vi "DriveBase.vi"(9 "Elevator State":string="Hatch_Rocket_1") -> ()   [LabVIEW 2018]
uses:
  RobotStates.vi
  Inputs_DriverStation.vi
  SensorReadings.vi
panel:
  in  "Forward Acceleration (p/s)":dbl=10.0
  in  "Time Above Speed (ms)":u32=100
  in  "Stabilization Height (in)":dbl=36.0
  in  "Switch to Low Gear (ft/s)":dbl=0.5
  in  "Switch to High Gear (ft/s)":dbl=5.0
  in  "Elevator Danger Height (in)":dbl=52.0
  in  "Backward Acceleration (p/s)":dbl=1.0
  in  "Climb-Drive Bias":dbl=-0.4
  in  "Turning Deadband":dbl=0.1
  in  "Throttle Deadband":dbl=0.2
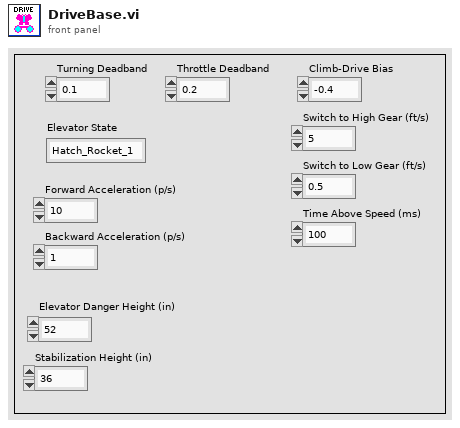
[diagram p1: front panel]
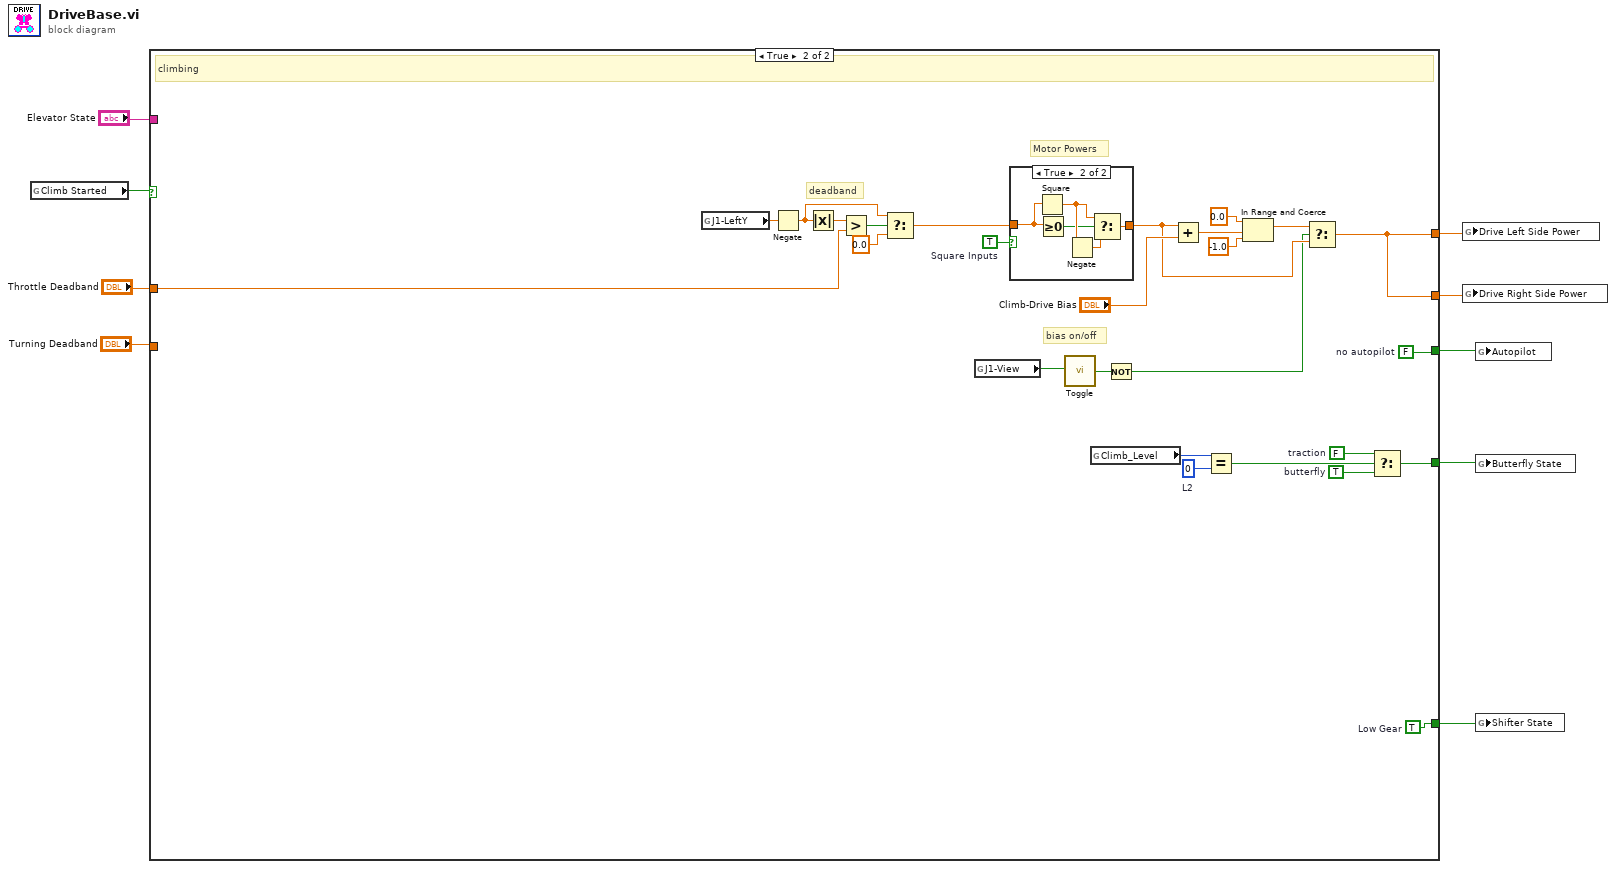
[diagram p0: block diagram]
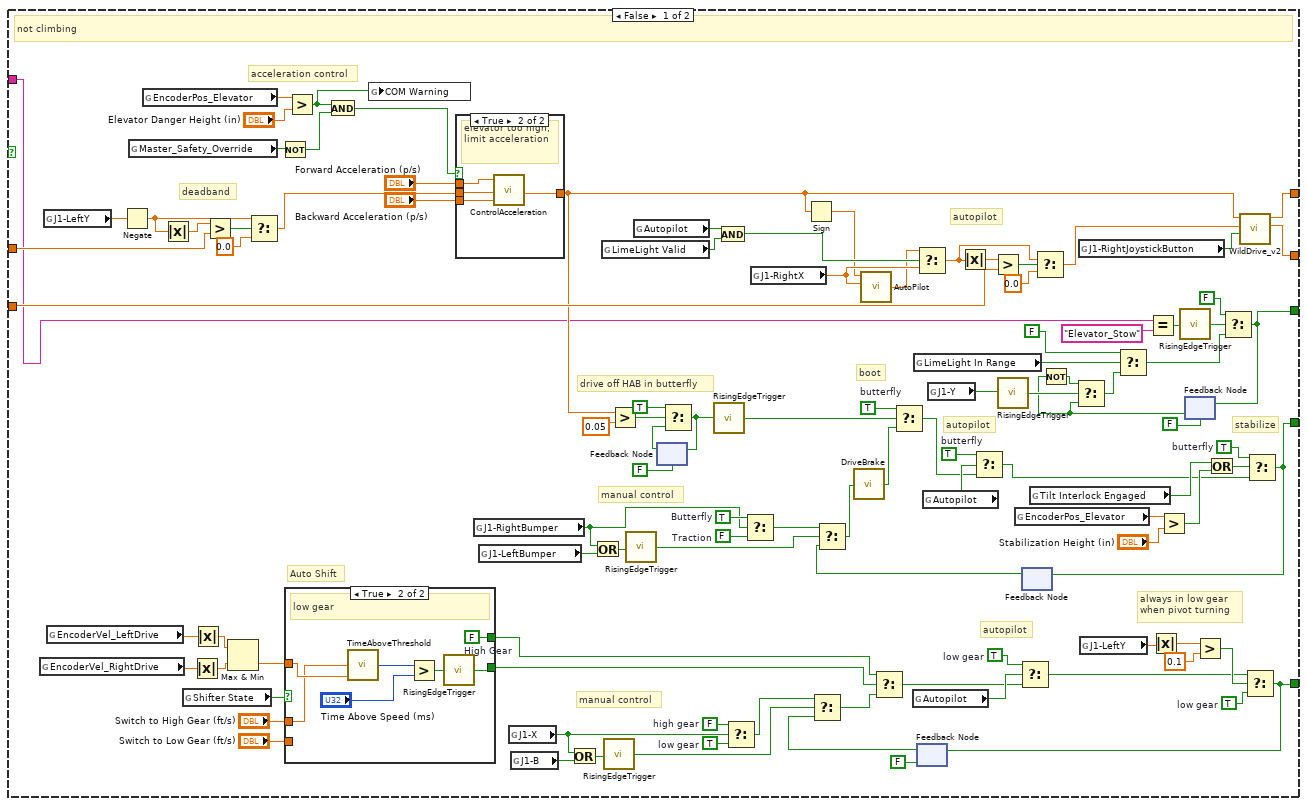
[diagram p2: hidden frame]
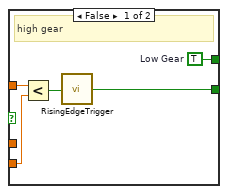
[diagram p3: hidden frame]
diagram:
  n1 = global read "RobotStates.vi" "Climb Started"() -> (w5:bool)
  n2 = case shown="True" w5 {
    tunnel: [w53 w137] -> w9
    tunnel: [w43 w157] -> w8
    tunnel: "Throttle Deadband" -> [w105 w149]
    tunnel: "Turning Deadband" -> [w104 _]
    tunnel: [w95 w139] -> w1
    tunnel: [w94 w139] -> w2
    tunnel: [w20 w138] -> w4
    tunnel: "Elevator State" -> [w19 _]
    frame False {
      w32 = TRUE  # butterfly
      w35 = TRUE  # low gear
      w42 = TRUE  # low gear
      w54 = FALSE  # Traction
      w55 = TRUE  # Butterfly
      w61 = TRUE  # butterfly
      w68 = TRUE  # butterfly
      w97 = TRUE  # low gear
      w98 = FALSE  # high gear
      # "deadband"
      # "acceleration control"
      # "always in low gear\nwhen pivot turning"
      # "autopilot"
      # "manual control"
      # "stabilize"
      # "autopilot"
      # "boot"
      # "manual control"
      # "autopilot"
      # "drive off HAB in butterfly"
      # "Auto Shift"
      # "not climbing"
      n3 = global read "SensorReadings.vi" "EncoderVel_RightDrive"() -> (w77:dbl)
      n4 = global read "Inputs_DriverStation.vi" "J1-LeftY"() -> (w110:dbl)
      n5 = global read "SensorReadings.vi" "EncoderVel_LeftDrive"() -> (w78:dbl)
      n6 = Negate(x=w110) -> (-x=w113:dbl)
      n7 = global read "Inputs_DriverStation.vi" "Master_Safety_Override"() -> (w83:bool)
      n8 = global read "SensorReadings.vi" "EncoderPos_Elevator"() -> (w86:dbl)
      n9 = Absolute Value(x=w113) -> (abs(x)=w108:dbl)
      n10 = global read "RobotStates.vi" "Shifter State"() -> (w76:bool)
      n11 = Absolute Value(x=w77) -> (abs(x)=w70:dbl)
      n12 = Absolute Value(x=w78) -> (abs(x)=w71:dbl)
      n13 = Greater?(x=w108, y=w105) -> (0:w109:bool)
      n14 = Max & Min(x=w71, y=w70) -> (min(x,y)=w49:dbl)  [unwired: 1 out]
      n15 = Select(t=w113, s=w109, f=0.0) -> (s? t:f=w88:dbl)
      n16 = Not(x=w83) -> (.not. x?=w82:bool)
      n17 = case shown="True" w76 {
        tunnel: w49 -> [w119 w121]
        tunnel: "Switch to High Gear (ft/s)" -> [_ w120]
        tunnel: "Switch to Low Gear (ft/s)" -> [w118 _]
        tunnel: [w115 w125] -> w69
        tunnel: [w117 w126] -> w72
        frame False {
          w117 = TRUE  # Low Gear
          # "high gear"
          n18 = Less?(x=w119, y=w118) -> (x < y?=w116:bool)
          n19 = call "RisingEdgeTrigger.vi"("Raw Signal"=w116) -> ("Trigger"=w115:bool)
        }
        frame True {
          w126 = FALSE  # High Gear
          # "low gear"
          n20 = call "TimeAboveThreshold.vi"("Current Value"=w121, "Threshold"=w120) -> ("Time Above"=w124:u32)  [unwired: 3 in]
          n21 = Greater?(x=w124, y="Time Above Speed (ms)") -> (0:w122:bool)
          n22 = call "RisingEdgeTrigger.vi"("Raw Signal"=w122) -> ("Trigger"=w125:bool)
        }
      }
      n23 = Greater?(x=w86, y="Elevator Danger Height (in)") -> (0:w79:bool)
      n24 = And(x=w79, y=w82) -> (x .and. y?=w84:bool)
      n25 = global write "RobotStates.vi" "COM Warning"(w79) -> ()
      n26 = case shown="True" w84 {
        tunnel: w88 -> [w127 w131]
        tunnel: [w127 w130] -> w29
        tunnel: "Backward Acceleration (p/s)" -> [_ w129]
        tunnel: "Forward Acceleration (p/s)" -> [_ w128]
        frame False {
          # "elevator down"
        }
        frame True {
          # "elevator too high, limit acceleration"
          n27 = call "ControlAcceleration.vi"("Backward Acceleration (p/s)"=w129, "Raw"=w131, "Forward Acceleration (p/s)"=w128) -> ("Controlled"=w130:dbl)
        }
      }
      n28 = global read "Inputs_DriverStation.vi" "J1-RightBumper"() -> (w51:bool)
      n29 = global read "Inputs_DriverStation.vi" "J1-LeftBumper"() -> (w52:bool)
      n30 = global read "Inputs_DriverStation.vi" "J1-X"() -> (w44:bool)
      n31 = global read "Inputs_DriverStation.vi" "J1-B"() -> (w102:bool)
      n32 = Or(x=w44, y=w102) -> (x .or. y?=w103:bool)
      n33 = Or(x=w51, y=w52) -> (x .or. y?=w59:bool)
      n34 = global read "SensorReadings.vi" "LimeLight Valid"() -> (w89:bool)
      n35 = call "RisingEdgeTrigger.vi"("Raw Signal"=w103) -> ("Trigger"=w99:bool)
      n36 = Greater?(x=w29, y=0.05) -> (0:w63:bool)
      n37 = call "RisingEdgeTrigger.vi"("Raw Signal"=w59) -> ("Trigger"=w56:bool)
      n38 = global read "RobotStates.vi" "Autopilot"() -> (w91:bool)
      n39 = feedback #1(FALSE) -> (w66:bool)
      n40 = Select(t=TRUE, s=w63, f=w66) -> (s? t:f=w65:bool)
      n41 = feedback-in #1(w65) -> ()
      n42 = call "RisingEdgeTrigger.vi"("Raw Signal"=w65) -> ("Trigger"=w50:bool)
      n43 = And(x=w91, y=w89) -> (x .and. y?=w90:bool)
      n44 = Select(t=w98, s=w44, f=w97) -> (s? t:f=w100:bool)
      n45 = Select(t=w55, s=w51, f=w54) -> (s? t:f=w57:bool)
      n46 = global read "Inputs_DriverStation.vi" "J1-RightX"() -> (w81:dbl)
      n47 = Sign(1:w29) -> (0:w28:dbl)
      n48 = call "AutoPilot.vi"("Human Contribution"=w81, "Drive Direction"=w28) -> ("End Contribution"=w80:dbl)  [unwired: 2 in]
      n49 = global read "RobotStates.vi" "Autopilot"() -> (w36:bool)
      n50 = global read "SensorReadings.vi" "LimeLight In Range"() -> (w12:bool)
      n51 = Select(t=w80, s=w90, f=w81) -> (s? t:f=w92:dbl)
      n52 = feedback #2(FALSE ("Low Gear")) -> (w101:bool)
      n53 = Select(t=w100, s=w99, f=w101) -> (s? t:f=w73:bool)
      n54 = Select(t=w72, s=w69, f=w73) -> (s? t:f=w34:bool)
      n55 = global read "RobotStates.vi" "Autopilot"() -> (w33:bool)
      n56 = global read "Inputs_DriverStation.vi" "J1-Y"() -> (w21:bool)
      n57 = Absolute Value(x=w92) -> (abs(x)=w111:dbl)
      n58 = Greater?(x=w111, y=w104) -> (0:w112:bool)
      n59 = call "RisingEdgeTrigger.vi"("Raw Signal"=w21) -> ("Trigger"=w24:bool)
      n60 = global read "SensorReadings.vi" "EncoderPos_Elevator"() -> (w48:dbl)
      n61 = Select(t=w35, s=w36, f=w34) -> (s? t:f=w37:bool)
      n62 = feedback #3() -> (w58:bool)  [unwired: 1 in]
      n63 = Select(t=w57, s=w56, f=w58) -> (s? t:f=w14:bool)
      n64 = call "DriveBrake.vi"("Butterfly State In"=w14) -> ("Butterfly State Out"=w15:bool)
      n65 = Select(t=w68, s=w50, f=w15) -> (s? t:f=w31:bool)
      n66 = Select(t=w32, s=w33, f=w31) -> (s? t:f=w30:bool)
      n67 = global read "RobotStates.vi" "Tilt Interlock Engaged"() -> (w45:bool)
      n68 = Select(t=w92, s=w112, f=0.0) -> (s? t:f=w114:dbl)
      n69 = global read "Inputs_DriverStation.vi" "J1-RightJoystickButton"() -> (w93:bool)
      n70 = global read "Inputs_DriverStation.vi" "J1-LeftY"() -> (w41:dbl)
      n71 = Equal?(x=w19, y="Elevator_Stow") -> (x = y?=w17:bool)
      n72 = Absolute Value(x=w41) -> (abs(x)=w40:dbl)
      n73 = Greater?(x=w48, y="Stabilization Height (in)") -> (0:w46:bool)
      n74 = call "RisingEdgeTrigger.vi"("Raw Signal"=w17) -> ("Trigger"=w16:bool)
      n75 = feedback #4(FALSE) -> (w22:bool)
      n76 = Not(x=w22) -> (.not. x?=w23:bool)
      n77 = Select(t=w23, s=w24, f=w22) -> (s? t:f=w11:bool)
      n78 = Select(t=FALSE, s=w12, f=w11) -> (s? t:f=w10:bool)
      n79 = Greater?(x=w40, y=0.1) -> (0:w39:bool)
      n80 = Or(x=w45, y=w46) -> (x .or. y?=w60:bool)
      n81 = Select(t=FALSE, s=w16, f=w10) -> (s? t:f=w20:bool)
      n82 = feedback-in #4(w20) -> ()
      n83 = call "WildDrive_v2.vi"("Super Turn"=w93, "Turn"=w114, "Speed"=w29) -> ("Right Side Power"=w94:dbl, "Left Side Power"=w95:dbl)  [unwired: 7 in]
      n84 = Select(t=w37, s=w39, f=w42) -> (s? t:f=w43:bool)
      n85 = feedback-in #2(w43) -> ()
      n86 = Select(t=w61, s=w60, f=w30) -> (s? t:f=w53:bool)
      n87 = feedback-in #3(w53) -> ()
    }
    frame True {
      w133 = u8 0  # L2
      w135 = FALSE  # traction
      w138 = FALSE  # no autopilot
      w151 = TRUE  # Square Inputs
      w157 = TRUE  # Low Gear
      w136 = TRUE  # butterfly
      # "deadband"
      # "bias on/off"
      # "Motor Powers"
      # "climbing"
      n88 = global read "Inputs_DriverStation.vi" "J1-LeftY"() -> (w154:dbl)
      n89 = Negate(x=w154) -> (-x=w155:dbl)
      n90 = Absolute Value(x=w155) -> (abs(x)=w152:dbl)
      n91 = Greater?(x=w152, y=w149) -> (0:w153:bool)
      n92 = Select(t=w155, s=w153, f=0.0) -> (s? t:f=w156:dbl)
      n93 = global read "Inputs_DriverStation.vi" "J1-View"() -> (w144:bool)
      n94 = case shown="True" w151 {
        tunnel: [w158 w163] -> w141
        tunnel: w156 -> [w158 w162]
        frame False {
        }
        frame True {
          n95 = Square(x=w162) -> (x^2=w160:dbl)
          n96 = Greater Or Equal To 0?(x=w162) -> (x >= 0?=w159:bool)
          n97 = Negate(x=w160) -> (-x=w161:dbl)
          n98 = Select(t=w160, s=w159, f=w161) -> (s? t:f=w163:dbl)
        }
      }
      n99 = call "Toggle.vi"("Trigger"=w144) -> ("New Mode"=w143:bool)
      n100 = global read "Inputs_DriverStation.vi" "Climb_Level"() -> (w134:u8)
      n101 = Not(x=w143) -> (.not. x?=w140:bool)
      n102 = Add(x=w141, y="Climb-Drive Bias") -> (x+y=w148:dbl)
      n103 = Equal?(x=w134, y=w133) -> (x = y?=w132:bool)
      n104 = In Range and Coerce(upper limit=0.0, x=w148, lower limit=-1.0) -> (coerced(x)=w142:dbl)  [unwired: 1 out]
      n105 = Select(t=w142, s=w140, f=w141) -> (s? t:f=w139:dbl)
      n106 = Select(t=w135, s=w132, f=w136) -> (s? t:f=w137:bool)
    }
  }
  n107 = global write "RobotStates.vi" "Drive Left Side Power"(w1) -> ()
  n108 = global write "RobotStates.vi" "Drive Right Side Power"(w2) -> ()
  n109 = global write "RobotStates.vi" "Autopilot"(w4) -> ()
  n110 = global write "RobotStates.vi" "Butterfly State"(w9) -> ()
  n111 = global write "RobotStates.vi" "Shifter State"(w8) -> ()
